vi "ConvertSampleMode.vi"(1 "SamplingMode":T1) -> (0 "sample mode":i32)   [LabVIEW 2020, in "DAQmx.AO.lvclass"]
uses:
  DAQmx.AO.lvclass
  DAQ/Typedefs/DAQ_SamplingMode.ctl
  DAQ/DAQ.lvclass
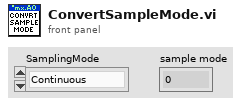
[diagram p1: front panel]
types:
  T1 = typedef "DAQ.lvclass/DAQ_SamplingMode.ctl" = enum16{"Continuous", "Finite"}
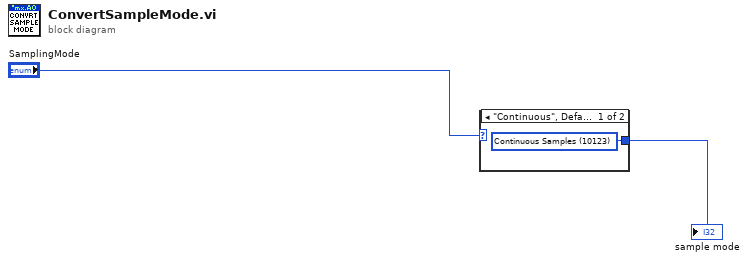
[diagram p0: block diagram]
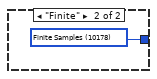
[diagram p2: hidden frame]
diagram:
  n1 = case shown="\"Continuous\", Default" "SamplingMode" {
    tunnel: [w3 w4] -> w2
    frame "Continuous", Default {
      w3 = 10123 items=["Finite Samples"=10178, "Continuous Samples"=10123, "Hardware Timed Single Point"=12522] ("sample mode")
    }
    frame "Finite" {
      w4 = 10178 items=["Finite Samples"=10178, "Continuous Samples"=10123, "Hardware Timed Single Point"=12522] ("sample mode")
    }
  }
  "sample mode" <- w2
